vi "ofdm_subcarrier_allocator.vi"(8 "fft size":u32=256, 9 "pilot symbol":cdb[](array[numeric]), 11 "message symbol":cdb[](array[numeric])) -> (3 "OFDM symbol":cdb[](array[numeric]))   [LabVIEW 2014]
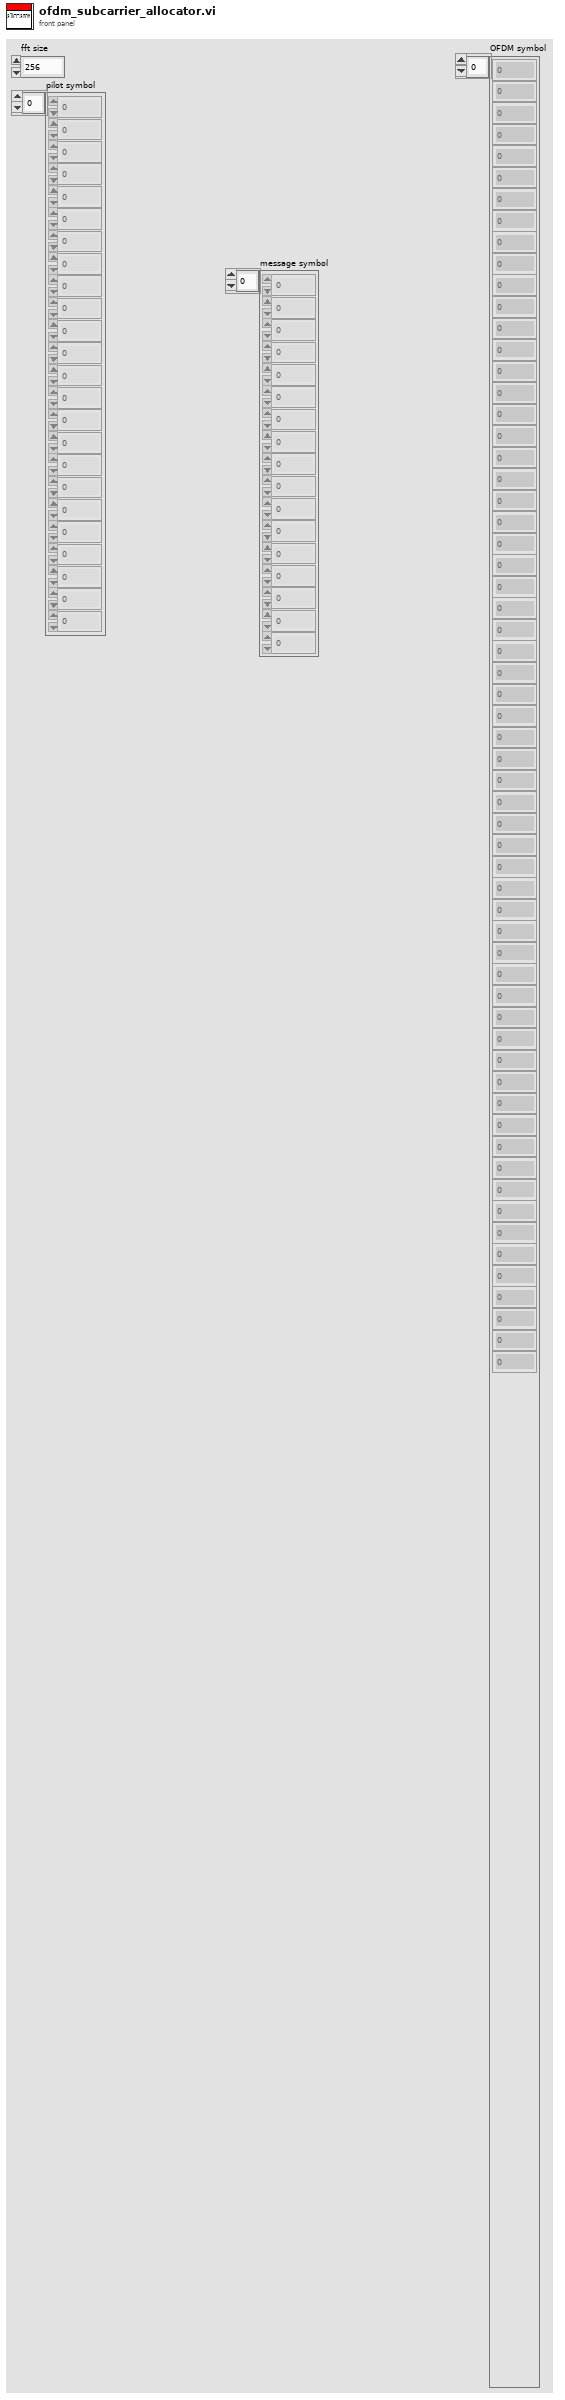
[diagram p1: front panel]
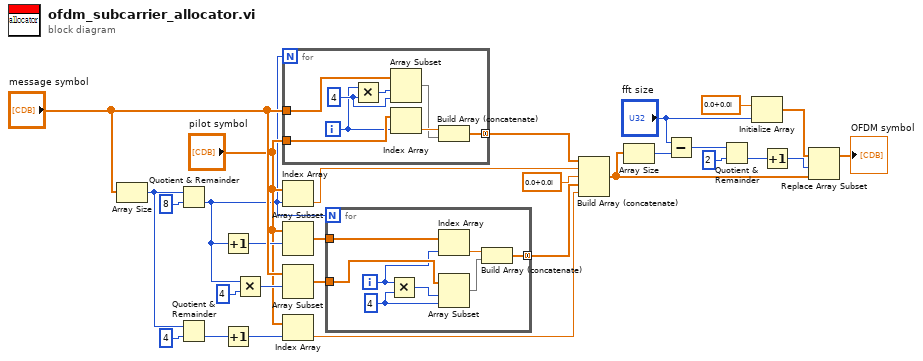
[diagram p0: block diagram]
diagram:
  n1 = Array Size(array="message symbol") -> (size(s)=w16:i32)
  n2 = Quotient & Remainder(x=w16, y=8) -> (floor(x/y)=w10:i32)  [unwired: 1 out]
  n3 = Quotient & Remainder(x=w16, y=4) -> (floor(x/y)=w11:i32)  [unwired: 1 out]
  n4 = Increment(x=w10) -> (x+1=w20:i32)
  n5 = Increment(x=w11) -> (x+1=w14:i32)
  n6 = Multiply(x=w10, y=4) -> (x*y=w22:i32)
  n7 = for {
    N: w10 -> [_]
    tunnel: "message symbol" -> [w34]
    tunnel: "pilot symbol" -> [w33]
    tunnel: [w29] -> w6 mode=concatenating
    i -> [w32]
    w36 = 4
    n8 = Multiply(x=w32, y=w36) -> (x*y=w35:i32)
    n9 = Array Subset(array=w34, index=w35, length=w36) -> (w30:cdb[])
    n10 = Index Array(array=w33, index=w32) -> (element=w31:cdb)
    n11 = Build Array (concatenate)(w31, w30) -> (w29:cdb[])
  }
  n12 = Index Array(array="pilot symbol", index=w10) -> (element=w26:cdb)
  n13 = Array Subset(array="pilot symbol", index=w20) -> (w19:cdb[])  [unwired: 1 in]
  n14 = Array Subset(array="message symbol", index=w22) -> (w21:cdb[])  [unwired: 1 in]
  n15 = Index Array(array="pilot symbol", index=w14) -> (element=w18:cdb)
  n16 = for {
    N: w10 -> [_]
    tunnel: w21 -> [w42]
    tunnel: w19 -> [w41]
    tunnel: [w37] -> w5 mode=concatenating
    i -> [w40]
    w44 = 4
    n17 = Multiply(x=w40, y=w44) -> (x*y=w43:i32)
    n18 = Index Array(array=w41, index=w40) -> (element=w39:cdb)
    n19 = Array Subset(array=w42, index=w43, length=w44) -> (w38:cdb[])
    n20 = Build Array (concatenate)(w39, w38) -> (w37:cdb[])
  }
  n21 = Build Array (concatenate)(w6, w26, cdb 0.0+0.0i, w5, w18) -> (w12:cdb[])
  n22 = Array Size(array=w12) -> (size(s)=w9:i32)
  n23 = Subtract(x="fft size", y=w9) -> (x-y=w8:u32)
  n24 = Quotient & Remainder(x=w8, y=2) -> (floor(x/y)=w4:u32)  [unwired: 1 out]
  n25 = Initialize Array(cdb 0.0+0.0i, "fft size") -> (w13:cdb[])
  n26 = Increment(x=w4) -> (x+1=w3:u32)
  n27 = Replace Array Subset(array=w13, new element=w12, index=w3) -> (→"OFDM symbol":cdb[])
